vi "SetDataTrProcMode.vi"(8 "错误输入（无错误）":errorcluster, 11 "数据传输模式":u8) -> (0 "错误输出":errorcluster)   [LabVIEW 2018]
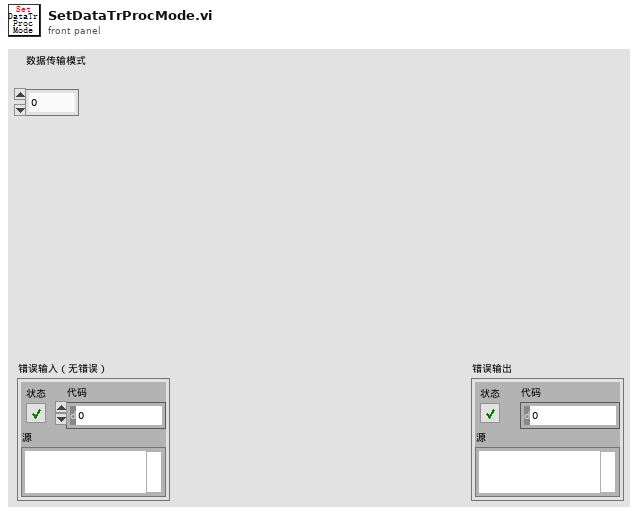
[diagram p1: front panel]
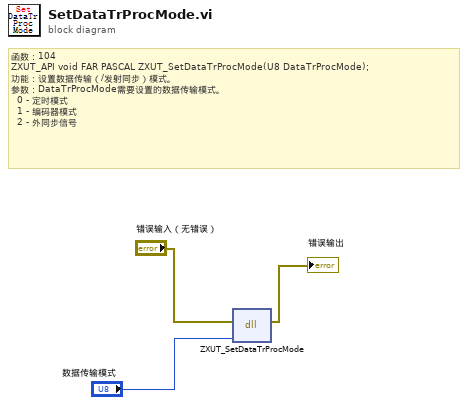
[diagram p0: block diagram]
diagram:
  # "函数：104\nZXUT_API void\tFAR PASCAL ZXUT_SetDataTrProcMode(U8 DataTrProcMode);\n功能：设置数据传输（/发射同步）模式。\n参数：DataTrProcMode需要设置的数据传输模式。\n\t\t0 - 定时模式\n\t\t1 - 编码器模式\n\t\t2 - 外同步信号"
  n1 = dll-call lib="PTH2Rabs E软件项目超声超声子VI函数VI\tTCG处理ZXUTConfigMgr.dll" fn="ZXUT_SetDataTrProcMode"(error in="错误输入（无错误）", "DataTrProcMode"="数据传输模式") -> (error out=→"错误输出":errorcluster)  [unwired: 4 in, 1 out]
